vi "CreateMap.vi"(11 "Mapping file path":path=path "C:/Users/deaton/Desktop/ECU Pin Mapping.csv") -> (0 "error out":errorcluster, 3 "LookupTable":refnum<data-value>)   [LabVIEW 2024, in "Shared Steps.lvlib"]
doc: "Load mapping file (CSV), create map, and create DVR reference to the map."
uses:
  Shared Steps.lvlib
  Types/Pin Mapping.ctl
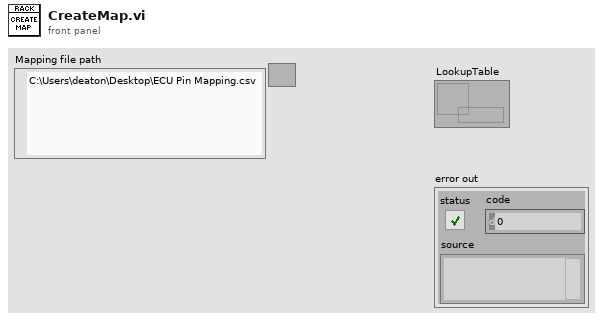
[diagram p1: front panel]
types:
  T1 = typedef "Shared Steps.lvlib/Pin Mapping.ctl" = cluster{"DUT":string, "ECU Pin Name":string, "Device Pin Name":string, "ECU Signal Type":string, "ECU Signal Direction":string, "MessageID":string}
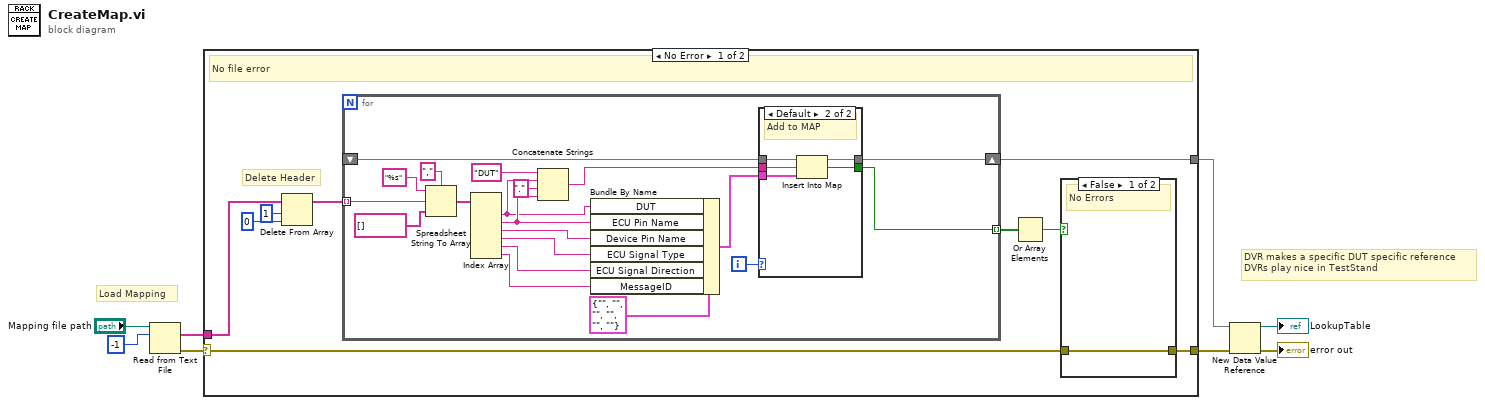
[diagram p0: block diagram]
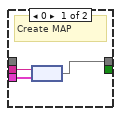
[diagram p2: hidden frame]
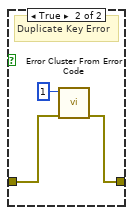
[diagram p3: hidden frame]
diagram:
  # "DVR makes a specific DUT specific reference\nDVRs play nice in TestStand"
  # "Load Mapping"
  n1 = Read from Text File(file (use dialog)="Mapping file path", count=-1) -> (text=w7:string[], error out=w5:errorcluster)  [unwired: 2 in, 2 out]
  n2 = case shown="No Error" w5 {
    selector: w5 -> [w13 w50]
    tunnel: w7 -> [w17 _]
    tunnel: [w11 w50] -> w3
    tunnel: [w10 _] -> w4
    frame No Error {
      # "Delete Header"
      # "No file error"
      n3 = Delete From Array(array=w17, length=1, index=0) -> (array with subset deleted=w14:string[])  [unwired: 1 out]
      n4 = for {
        shift-right: [w36] -> w10
        shift-left: _ -> [w37]
        tunnel: [w35] -> w16 mode=indexing
        tunnel: w14 -> [w30] mode=indexing
        i -> [w29]
        n5 = Spreadsheet String To Array(delimiter (Tab)=",", format string="%s" ("spreadsheet string"), spreadsheet string=w30, array type (2D Dbl)=string[] []) -> (array=w32:string[])
        n6 = Index Array(array=w32) -> (element #1=w18:string, element #2=w19:string, element #3=w23:string, element #4=w24:string, element #5=w25:string, element #6=w26:string)  [unwired: 6 in]
        n7 = Concatenate Strings("DUT" ("string"), w18, "." ("string"), w19) -> (w21:string)
        n8 = Bundle By Name(cluster=T1 {"DUT"="", "ECU Pin Name"="", "Device Pin Name"="", "ECU Signal Type"="", "ECU Signal Direction"="", "MessageID"=""}, "DUT"=w18, "ECU Pin Name"=w19, "Device Pin Name"=w23, "ECU Signal Type"=w24, "ECU Signal Direction"=w25, "MessageID"=w26) -> (w28:T1)
        n9 = case shown="Default" w29 {
          tunnel: w37 -> [_ w45]
          tunnel: [w38 w44] -> w36
          tunnel: [_ w43] -> w35
          tunnel: w21 -> [w40 w42]
          tunnel: w28 -> [w39 w41]
          frame 0 {
            # "Create MAP"
            n10 = node(w40, w39) -> (w38:map{string, T1})
          }
          frame Default {
            # "Add to MAP"
            n11 = Insert Into Map(map in=w45, key=w42, value=w41) -> (map out=w44:map{string, T1}, key already included?=w43:bool)  [unwired: 1 out]
          }
        }
      }
      n12 = Or Array Elements(Boolean array=w16) -> (logical OR=w12:bool)
      n13 = case shown="False" w12 {
        tunnel: w13 -> [w46 w48]
        tunnel: [w46 w47] -> w11
        frame False {
          # "No Errors"
        }
        frame True {
          # "Duplicate Key Error"
          n14 = call <vilib>:"Error Cluster From Error Code.vi"("error in (no error)"=w48, "error code (0)"=1) -> ("error out"=w47:errorcluster)  [unwired: 7 in]
        }
      }
    }
    frame Error {
      # "File Error"
    }
  }
  n15 = New Data Value Reference(data value=w4, error in=w3) -> (data value reference=→"LookupTable":refnum<data-value>, error out=→"error out":errorcluster)
